vi "nominal_channel_writer.write_data_cluster.vi"(6 "tags":map{string, string}(c390), 8 "error in":errorcluster, 9 "Custom Cluster Streamer":refnum<class "stream_custom_cluster.lvclass">, 10 "Data Source RID":string, 11 "Nominal Client in":refnum<class "Nominal Client.lvclass">) -> (0 "error out":errorcluster, 3 "Nominal Client out":refnum<class "Nominal Client.lvclass">, 4 "Terminated":bool)   [LabVIEW 2020, in "Nominal Client.lvclass"]
doc: "Synchronously writes a data cluster of records to a Nominal data source.\nSee `Streaming Cluster Data` example for useage notes."
uses:
  Nominal Client.lvclass
  Nominal Client.lvclass/Nominal Client.ctl
  stream_custom_cluster/stream_custom_cluster.lvclass
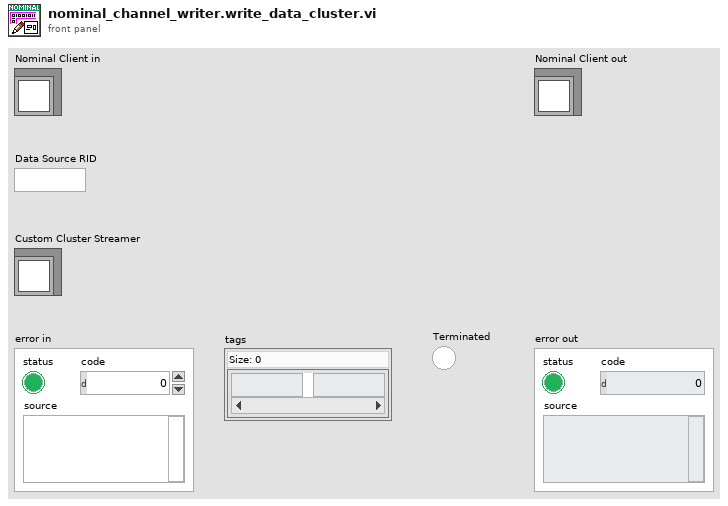
[diagram p1: front panel]
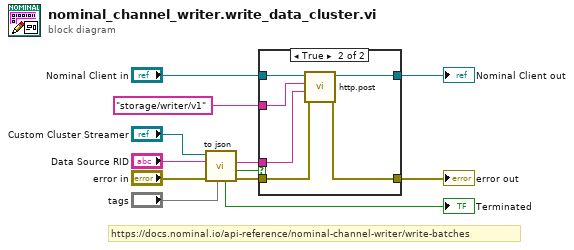
[diagram p0: block diagram]
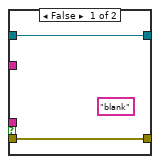
[diagram p2: hidden frame]
diagram:
  # "https://docs.nominal.io/api-reference/nominal-channel-writer/write-batches"
  n1 = call "to json.vi"("tags"="tags", "error in"="error in", "dataSourceRid"="Data Source RID", "stream_custom_cluster in"="Custom Cluster Streamer") -> ("error out"=w8:errorcluster, "Contains Data"=w3:bool, "json"=w4:string, "Terminated"=→"Terminated":bool)  [unwired: 3 in, 1 out]
  n2 = case shown="True" w3 {
    tunnel: "Nominal Client in" -> [w14 w20]
    tunnel: [w14 w19] -> w11
    tunnel: [w13 w18] -> w10
    tunnel: "storage/writer/v1" ("Path") -> [_ w17]
    tunnel: w8 -> [w13 w16]
    tunnel: w4 -> [_ w15]
    frame False {
      (unwired) "blank" ("json")
    }
    frame True {
      n3 = call "http.post.vi"("error in"=w16, "Request body"=w15, "Path"=w17, "Nominal Client in"=w20) -> ("error out"=w18:errorcluster, "Nominal Client out"=w19:refnum<class "Nominal Client.lvclass">)  [unwired: 5 in, 1 out]
    }
  }
  "Nominal Client out" <- w11
  "error out" <- w10
